vi "Reset Meas v 3.vi"(11 "simulate":bool) -> ()   [LabVIEW 2013]
panel:
  out "Loop Time":dbl
  out "Message":string
  in  "End Reset Routine":bool
  # "RESET BUSY"
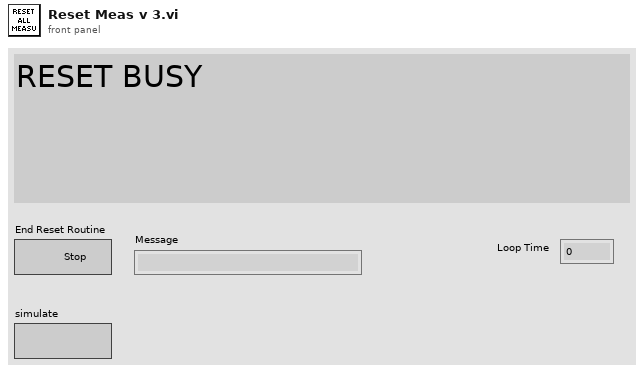
[diagram p1: front panel]
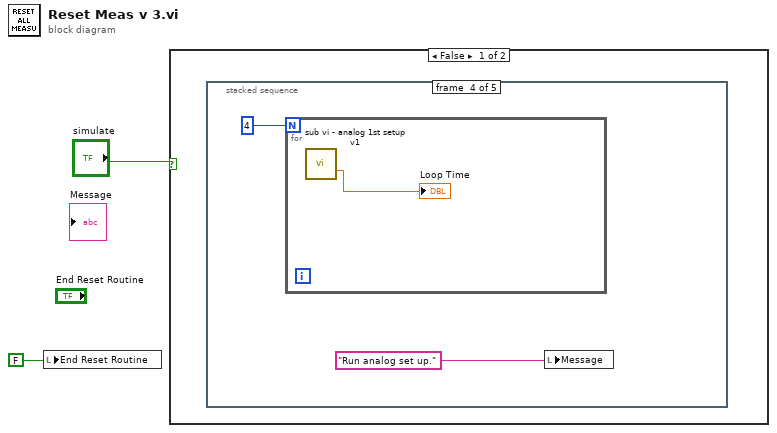
[diagram p0: block diagram]
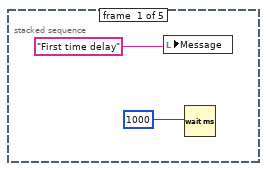
[diagram p2: hidden frame]
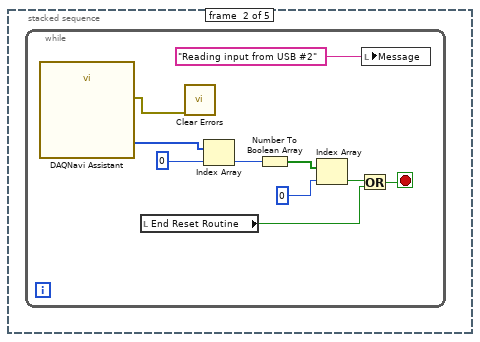
[diagram p3: hidden frame]
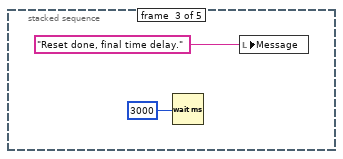
[diagram p4: hidden frame]
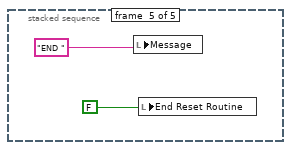
[diagram p5: hidden frame]
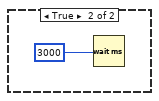
[diagram p6: hidden frame]
diagram:
  n1 = local write "End Reset Routine"(FALSE) -> ()
  n2 = case shown="False" "simulate" {
    frame False {
      n3 = stacked-sequence {
        frame #0 {
          n4 = local write "Message"("First time delay") -> ()
          n5 = Wait (ms)(milliseconds to wait=1000) -> ()  [unwired: 1 out]
        }
        frame #1 {
          n6 = while {
            stop <- w9 stop-if-true
            n7 = call "DAQNavi Assistant"() -> ("error out"=w7:errorcluster, "dataOut(U8Array)"=w10:u8[])  [unwired: 26 in]
            n8 = local read "End Reset Routine"() -> (w5:bool)
            n9 = call <vilib>:"Clear Errors.vi"("error in (no error)"=w7) -> ()  [unwired: 6 in, 1 out]
            n10 = Index Array(array=w10, index=0) -> (element=w12:u8)
            n11 = Number To Boolean Array(number=w12) -> (Boolean array=w13:bool[])
            n12 = Index Array(array=w13, index=0) -> (element=w8:bool)
            n13 = Or(x=w8, y=w5) -> (x .or. y?=w9:bool)
            n14 = local write "Message"("Reading input from USB #2") -> ()
          }
        }
        frame #2 {
          n15 = Wait (ms)(milliseconds to wait=3000) -> ()  [unwired: 1 out]
          n16 = local write "Message"("Reset done, final time delay.") -> ()
        }
        frame #3 {
          n17 = for {
            N: 4 -> [_]
            n18 = call "sub vi - analog 1st setup v1.vi"() -> ("loop time"=→"Loop Time":dbl)  [unwired: 9 in, 6 out]
          }
          n19 = local write "Message"("Run analog set up.") -> ()
        }
        frame #4 {
          n20 = local write "Message"("END ") -> ()
          n21 = local write "End Reset Routine"(FALSE) -> ()
        }
      }
    }
    frame True {
      n22 = Wait (ms)(milliseconds to wait=3000) -> ()  [unwired: 1 out]
    }
  }
